vi "RS232 Device.vi"(8 "error in (no error)":errorcluster) -> (0 "error out":errorcluster, 3 "COM":refnum<visa-resource-name>)   [LabVIEW 2013]
uses:
  <vilib>/Utility/config.llb/Write Key (String).vi
  <vilib>/Utility/config.llb/Read Key (String).vi
  <vilib>/Utility/config.llb/NI_LVConfig.lvlib
panel:
  out "COM Array":refnum<visa-resource-name>[](array[refnum])
  out "appended path":path
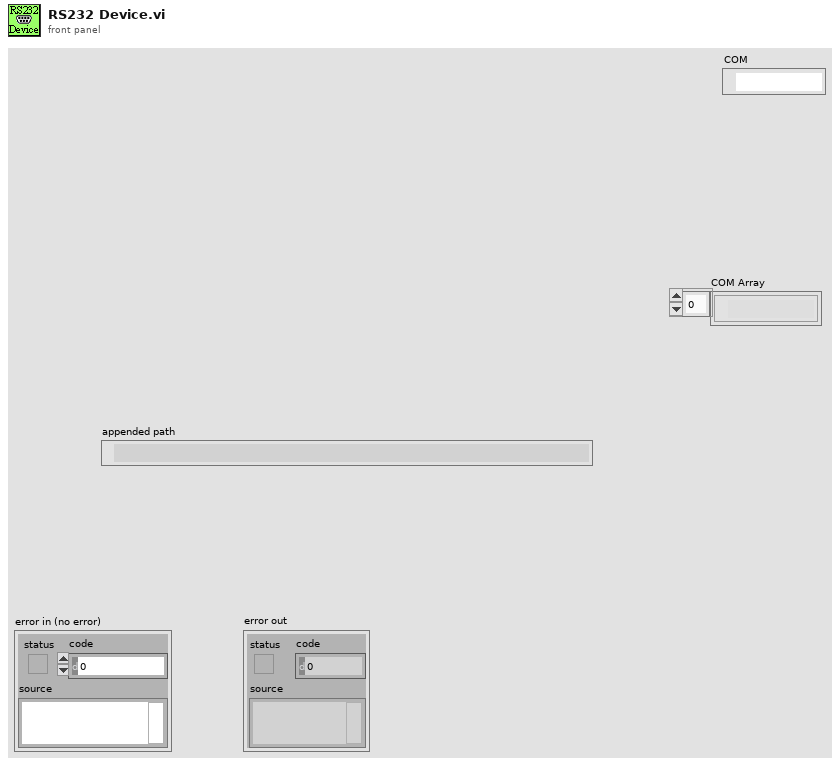
[diagram p1: front panel]
types:
  T1 = typedef "NI_LVConfig.lvlib/Config Data RefNum.ctl" = refnum<k1>
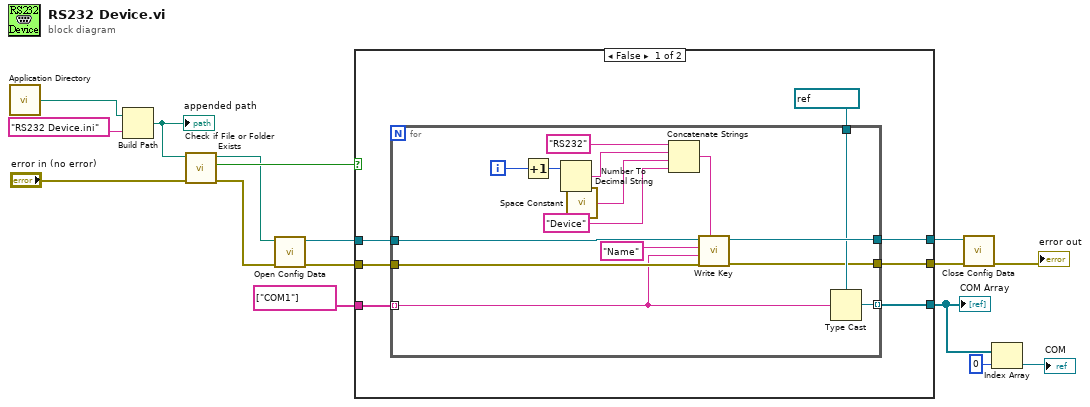
[diagram p0: block diagram]
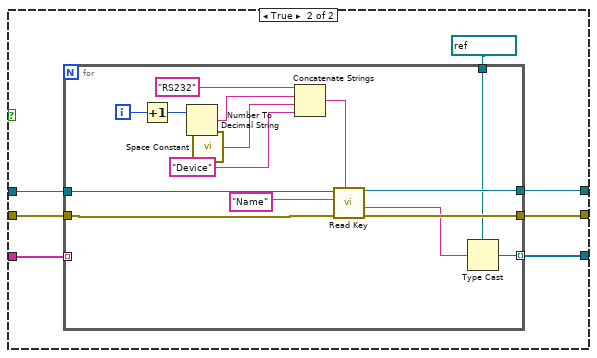
[diagram p2: hidden frame]
diagram:
  n1 = call <vilib>:"Application Directory.vi"() -> ("Application Directory"=w13:path)
  n2 = Build Path(base path=w13, name or relative path="RS232 Device.ini") -> (appended path=w15:path)
  "appended path" <- w15
  n3 = call <vilib>:"Check if File or Folder Exists.vi"("error in (no error)"="error in (no error)", "path"=w15) -> ("error out"=w5:errorcluster, "file or folder exists?"=w7:bool, "dup path"=w6:path)  [unwired: 7 in]
  n4 = call <vilib>:"Open Config Data.vi"("error in (no error)"=w5, "configuration file path"=w6) -> ("error out"=w10:errorcluster, "refnum"=w12:T1)  [unwired: 7 in, 1 out]
  n5 = case shown="False" w7 {
    tunnel: w12 -> [w23 w45]
    tunnel: [w22 w43] -> w11
    tunnel: w10 -> [w21 w42]
    tunnel: [w20 w44] -> w8
    tunnel: string[] ["COM1"] -> [w19 w41]
    tunnel: [w17 w39] -> w3
    frame False {
      n6 = for {
        tunnel: w23 -> [w38]
        tunnel: [w31] -> w22
        tunnel: refnum<visa-resource-name> "COM1" ("VISA resource name") -> [w30]
        tunnel: [w29] -> w17 mode=indexing
        tunnel: w21 -> [w28]
        tunnel: [w27] -> w20
        tunnel: w19 -> [w24] mode=indexing
        i -> [w26]
        n7 = Increment(x=w26) -> (x+1=w25:i32)
        n8 = Number To Decimal String(number=w25) -> (decimal integer string=w35:string)  [unwired: 1 in]
        n9 = call <vilib>:"Space Constant.vi"() -> ("String"=w36:string)
        n10 = Concatenate Strings("RS232" ("section"), w35, w36, "Device" ("section")) -> (w32:string)
        n11 = call-poly <vilib>:"Write Key.vi"("section"=w32, "error in (no error)"=w28, "value"=w24, "key"="Name", "refnum"=w38) -> ("error out"=w27:errorcluster, "refnum out"=w31:T1)  [unwired: 4 in, 1 out]
        n12 = Type Cast(type=w30, x=w24) -> (*(type *) &x=w29:refnum<visa-resource-name>)
      }
    }
    frame True {
      n13 = for {
        tunnel: w45 -> [w55]
        tunnel: [w52] -> w44
        tunnel: [w51] -> w43
        tunnel: [w49] -> w39 mode=indexing
        tunnel: refnum<visa-resource-name> "COM1" ("VISA resource name") -> [w46]
        tunnel: w42 -> [w48]
        tunnel: w41 -> [_] mode=indexing
        i -> [w57]
        n14 = Increment(x=w57) -> (x+1=w56:i32)
        n15 = Number To Decimal String(number=w56) -> (decimal integer string=w59:string)  [unwired: 1 in]
        n16 = call <vilib>:"Space Constant.vi"() -> ("String"=w58:string)
        n17 = Concatenate Strings("RS232" ("section"), w59, w58, "Device" ("section")) -> (w54:string)
        n18 = call-poly <vilib>:"Read Key.vi"("section"=w54, "error in (no error)"=w48, "key"="Name", "refnum"=w55) -> ("error out"=w52:errorcluster, "value"=w50:string, "refnum out"=w51:T1)  [unwired: 4 in, 1 out]
        n19 = Type Cast(type=w46, x=w50) -> (*(type *) &x=w49:refnum<visa-resource-name>)
      }
    }
  }
  "COM Array" <- w3
  n20 = call <vilib>:"Close Config Data.vi"("error in (no error)"=w8, "refnum"=w11) -> ("error out"=→"error out":errorcluster)  [unwired: 8 in, 1 out]
  n21 = Index Array(array=w3, index=0) -> (element=→"COM":refnum<visa-resource-name>)
